vi "Generate 1D Motion Profile Method 2.vi"(0 "Target Position":dbl=60.0, 1 "Initial Velocity (0)":dbl format="%#_13g", 3 "Final Velocity (0)":dbl format="%#_13g", 5 "Initial Position (0)":dbl format="%#_13g", 7 "Max Velocity":dbl=75.0, 9 "Max Acceleration":dbl=400.0, 11 "Error In":errorcluster, 12 "dt (.005)":dbl=0.005 format="%#_13g") -> (4 "Profile Plot":T1, 15 "Error Out":errorcluster)   [LabVIEW 2015]
uses:
  Typedef/Motion Profile.ctl
  <vilib>/Analysis/1siggen.llb/Ramp Pattern by Delta.vi
  <vilib>/Analysis/NI_AALPro.lvlib
  <vilib>/Analysis/NI_AALBase.lvlib
panel:
  out "XY Graph":cluster{"dX/dt":dbl[], "Ramp Pattern":dbl[]}[](graph)
  out "Total Time":dbl=nan
  in  "Max Jerk":dbl=5000.0
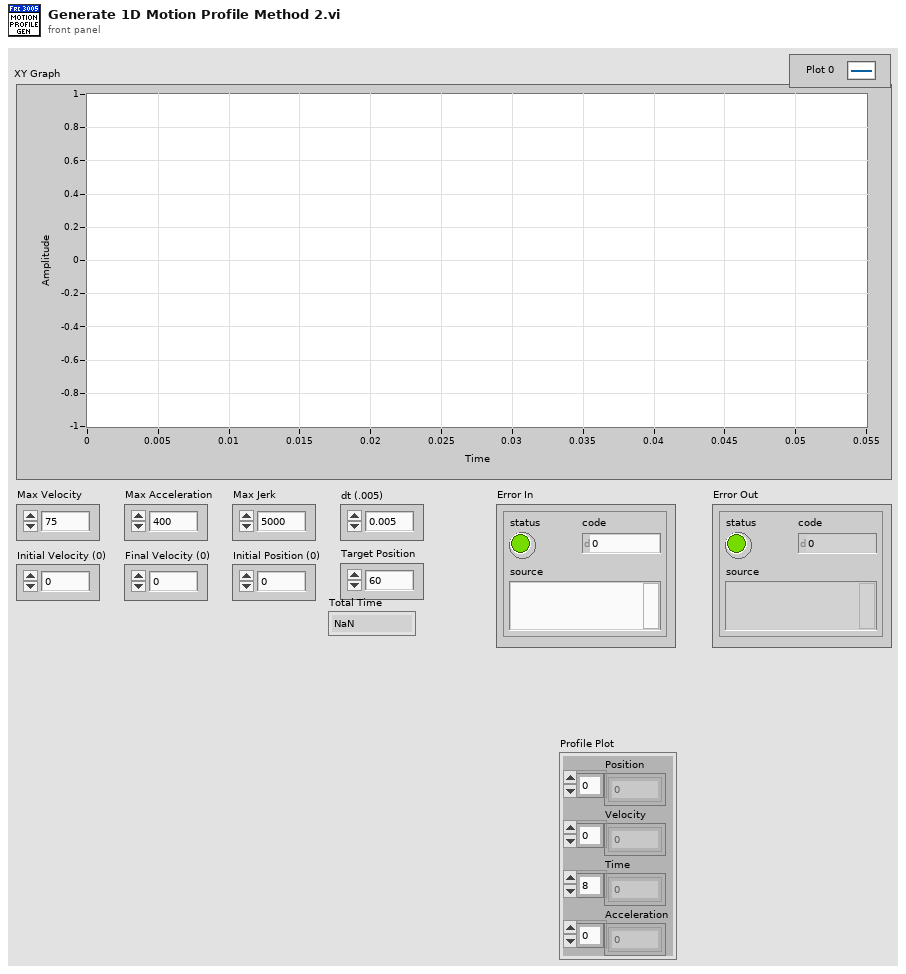
[diagram p1: front panel]
types:
  T1 = typedef "Motion Profile.ctl" = cluster{"Position":dbl[], "Velocity":dbl[], "Time":dbl[], "Acceleration":dbl[]}
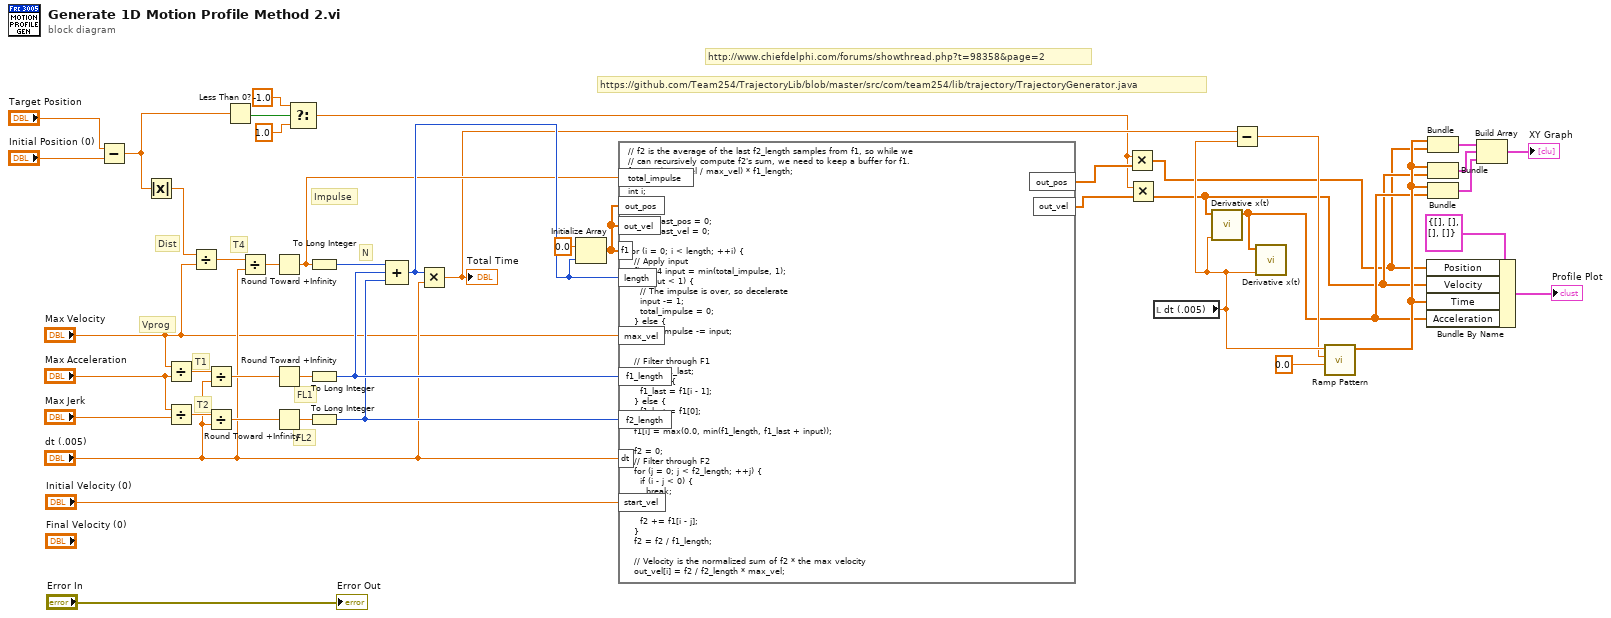
[diagram p0: block diagram]
diagram:
  # "https://github.com/Team254/TrajectoryLib/blob/master/src/com/team254/lib/trajectory/TrajectoryGenerator.java"
  # "Impulse"
  # "http://www.chiefdelphi.com/forums/showthread.php?t=98358&page=2"
  # "N"
  # "Dist"
  # "Vprog"
  # "T2"
  # "T1"
  # "T4"
  # "FL2"
  # "FL1"
  n1 = Subtract(x="Target Position", y="Initial Position (0)") -> (x-y=w8:dbl)
  n2 = Absolute Value(x=w8) -> (abs(x)=w7:dbl)
  n3 = Divide(x="Max Velocity", y="Max Acceleration") -> (x/y=w45:dbl)
  n4 = Divide(x="Max Acceleration", y="Max Jerk") -> (x/y=w44:dbl)
  n5 = Divide(x=w7, y="Max Velocity") -> (x/y=w41:dbl)
  n6 = Divide(x=w45, y="dt (.005)") -> (x/y=w39:dbl)
  n7 = Divide(x=w44, y="dt (.005)") -> (x/y=w38:dbl)
  n8 = Less Than 0?(x=w8) -> (x < 0?=w4:bool)
  n9 = Divide(x=w41, y="dt (.005)") -> (x/y=w40:dbl)
  n10 = Round Toward +Infinity(x=w40) -> (ceil(x): smallest int >= x=w30:dbl)
  n11 = Round Toward +Infinity(x=w39) -> (ceil(x): smallest int >= x=w35:dbl)
  n12 = Round Toward +Infinity(x=w38) -> (ceil(x): smallest int >= x=w36:dbl)
  n13 = Select(t=-1.0, s=w4, f=1.0) -> (s? t:f=w1:dbl)
  n14 = To Long Integer(number=w30) -> (32bit integer=w32:i32)
  n15 = To Long Integer(number=w35) -> (32bit integer=w29:i32)
  n16 = To Long Integer(number=w36) -> (32bit integer=w28:i32)
  n17 = Compound Arithmetic op=ADD(w32, w29, w28) -> (w31:i32)
  n18 = Multiply(x=w31, y="dt (.005)") -> (x*y=w20:dbl)
  "Total Time" <- w20
  n19 = Initialize Array(0.0 ("element"), w31) -> (w22:dbl[])
  n20 = formula code="// f2 is the average of the last f2_length samples from f1, so while we\n// can recursively compute f2's sum, we need to keep a buffer for f1.\nf1[0] = (start_vel / max_vel) * f1_length;\nfloat64 f2;\nint i;\nint j;\n\nfloat64 last_pos = 0;\nfloat64 last_vel = 0;\n\nfor (i = 0; i < length; ++i) {\n  // Apply input\n  float64 input = min(total_impulse, 1);\n  if (input < 1) {\n    // The impulse is over, so decelerate\n    input -= 1;\n    total_impulse = 0;\n  } else {\n    total_impulse -= input;\n  }\n\n  // Filter through F1\n  float64 f1_last;\n  if (i > 0) {\n    f1_last = f1[i - 1];\n  } else {\n    f1_last = f1[0];\n  }\n  f1[i] = max(0.0, min(f1_length, f1_last + input));\n\n  f2 = 0;\n  // Filter through F2\n  for (j = 0; j < f2_length; ++j) {\n    if (i - j < 0) {\n      break;\n    }\n\n    f2 += f1[i - j];\n  }\n  f2 = f2 / f1_length;\n\n  // Velocity is the normalized sum of f2 * the max velocity\n  out_vel[i] = f2 / f2_length * max_vel;\n  \n  out_pos[i] = (last_vel + out_vel[i]) / 2.0 * dt + last_pos;\n  \n  last_vel = out_vel[i];\n  last_pos = out_pos[i];\n}"("f1_length"=w29, "f2_length"=w28, "dt"="dt (.005)", "start_vel"="Initial Velocity (0)", "max_vel"="Max Velocity", "total_impulse"=w30, "length"=w31, "f1"=w22, "out_vel"=w22, "out_pos"=w22) -> ("out_vel"=w13:dbl[], "out_pos"=w14:dbl[])
  n21 = Multiply(x=w1, y=w14) -> (x*y=w5:dbl[])
  n22 = Multiply(x=w1, y=w13) -> (x*y=w6:dbl[])
  n23 = local read "dt (.005)"() -> (w19:dbl)
  n24 = call <vilib>:"Derivative x(t).vi"("dt"=w19, "X"=w6) -> ("dX/dt"=w12:dbl[])  [unwired: 8 in, 1 out]
  n25 = Subtract(x=w20, y=w19) -> (x-y=w18:dbl)
  n26 = call <vilib>:"Derivative x(t).vi"("dt"=w19, "X"=w12) -> ()  [unwired: 8 in, 2 out]
  n27 = call-poly <vilib>:"Ramp Pattern.vi"("start"=0.0, "end"=w18, "delta"=w19) -> ("Ramp Pattern"=w17:dbl[])  [unwired: 6 in, 2 out]
  n28 = Bundle By Name(cluster=T1 {"Position"=[], "Velocity"=[], "Time"=[], "Acceleration"=[]} ("Profile Plot"), "Position"=w5, "Velocity"=w6, "Time"=w17, "Acceleration"=w12) -> (→"Profile Plot":T1)
  n29 = Bundle("Ramp Pattern"=w17, w5) -> (w16:cluster{"Ramp Pattern":dbl[], dbl[]})  [unwired: 1 in]
  n30 = Bundle("Ramp Pattern"=w17, w6) -> (w15:cluster{"Ramp Pattern":dbl[], dbl[]})  [unwired: 1 in]
  n31 = Bundle("Ramp Pattern"=w17, "dX/dt"=w12) -> (w24:cluster{"Ramp Pattern":dbl[], "dX/dt":dbl[]})  [unwired: 1 in]
  n32 = Build Array(w16, w15, w24) -> (→"XY Graph":cluster{"Ramp Pattern":dbl[], "dX/dt":dbl[]}[])
  "Error Out" <- "Error In"
